vi "HAPS_PhaseSweep.vi"() -> ()   [LabVIEW 2023, in "HAPS.lvlib"]
uses:
  HAPS.lvlib
  MCU_Function.ctl
  set_ele.ctl
  HAPS_SerialPort.ctl
  HAPS_MCU_ELE_Func.ctl
panel:
  in  "comn_gain":i32=17
  in  "ele_gain":i32=35
  in  "File_note":string
  in  "Init?":bool
  out "Duration":dbl
  out "In-Phase : Phase(degree)":dbl[](graph)
  out "In-Phase : Gain(dB)":dbl[](graph)
  out "channel":i32
  out "chain_id":i32
  out "group":i32
  out "array_id":i32
  in  "Phase diff. Criteria":dbl format="%#_13g"
  in  "Tx/Rx":enum16{"Rx", "Tx"}(ring)=enum."Tx"
  in  "array_id (MCU index)":i32
  in  "MCU_UART_addr":refnum<visa-resource-name>="COM1"
  in  "Target(degree)":dbl format="%#_13g"
  in  "SweepPoints":i32=11
  in  "sParameter":i32=21
  in  "Stop_Freq(GHz)":dbl=39.5
  in  "Start_Freq(GHz)":dbl=38.5
  in  "VISA resource name":refnum<visa-resource-name>="TCPIP0::169.254.52.242::hislip0::INSTR"
  in  "HAPS_Equipment":enum16{"Keysight", "R&S"}(ring)
  # "HAPS_24x24_Phase_Sweep"
  # "VNA"
  # "Tx:35\nRx:22"
  # "DUT"
  # "4718.54"
  # "TCPIP0::192.168.1.31::hislip0::INSTR"
  # "Test Status"
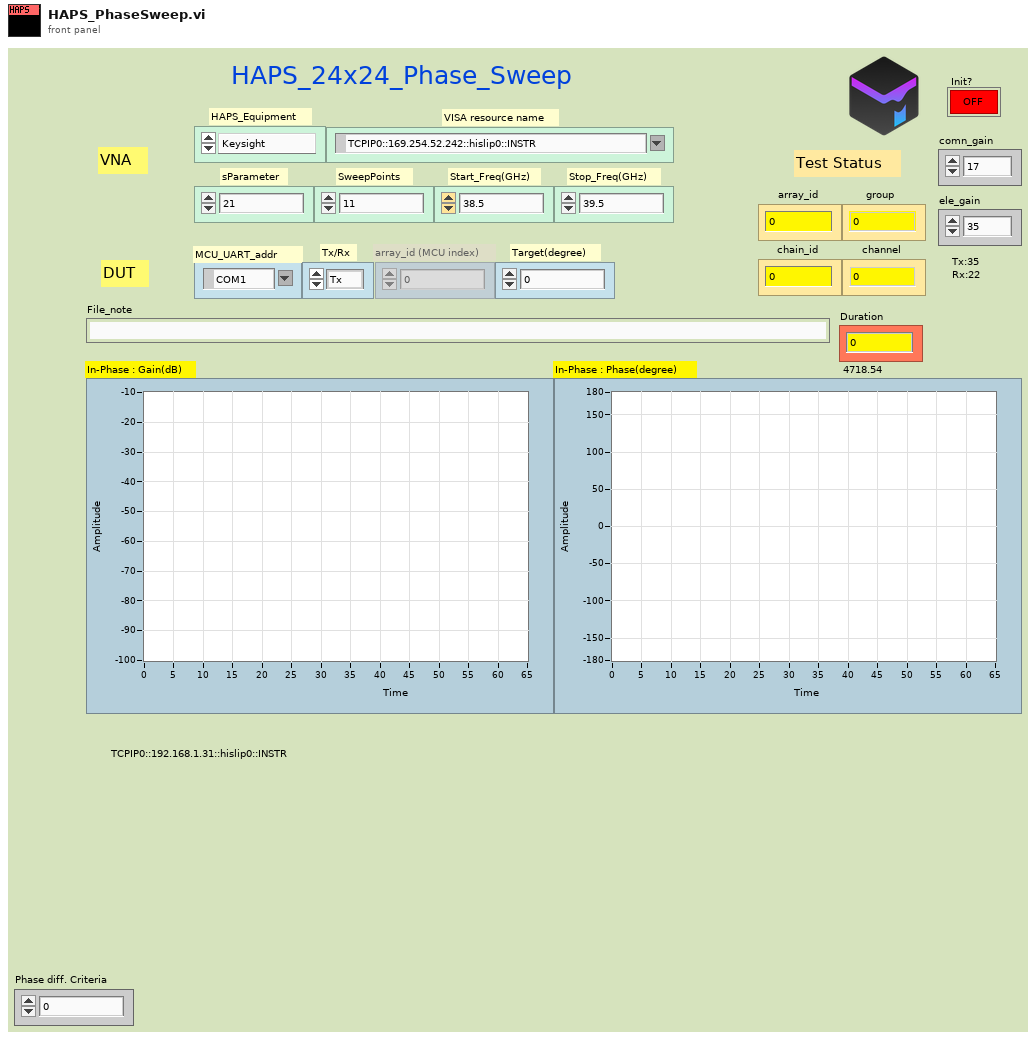
[diagram p1: front panel]
types:
  T1 = typedef "HAPS.lvlib/HAPS_SerialPort.ctl" = enum16{"Init", "Close", "CMD", "Flush"}
  T2 = typedef "HAPS.lvlib/HAPS_MCU_ELE_Func.ctl" = enum16{"array_init", "set_com_gain", "set_ch_gain_phase", "set_pd_range", "get_preamp_temp", "get_bfic_temp", "get_tx_pd", "ch_on", "ch_on_2", "ch_ctrl_all", "array_ctrl_src"}
  T3 = typedef "HAPS.lvlib/MCU_Function.ctl" = cluster{"Tx/Rx":enum16{"Rx", "Tx"}, "Enable?":enum16{"OFF", "On"}, "Source":enum16{"MCU", "ACU"}}
  T4 = typedef "HAPS.lvlib/set_ele.ctl" = cluster{"ch":i32, "chain_id":i32, "group":i32, "array_id":i32, "ele_phase":i32, "ele_gain":i32, "com_gain":i32, "pd_range":i32}
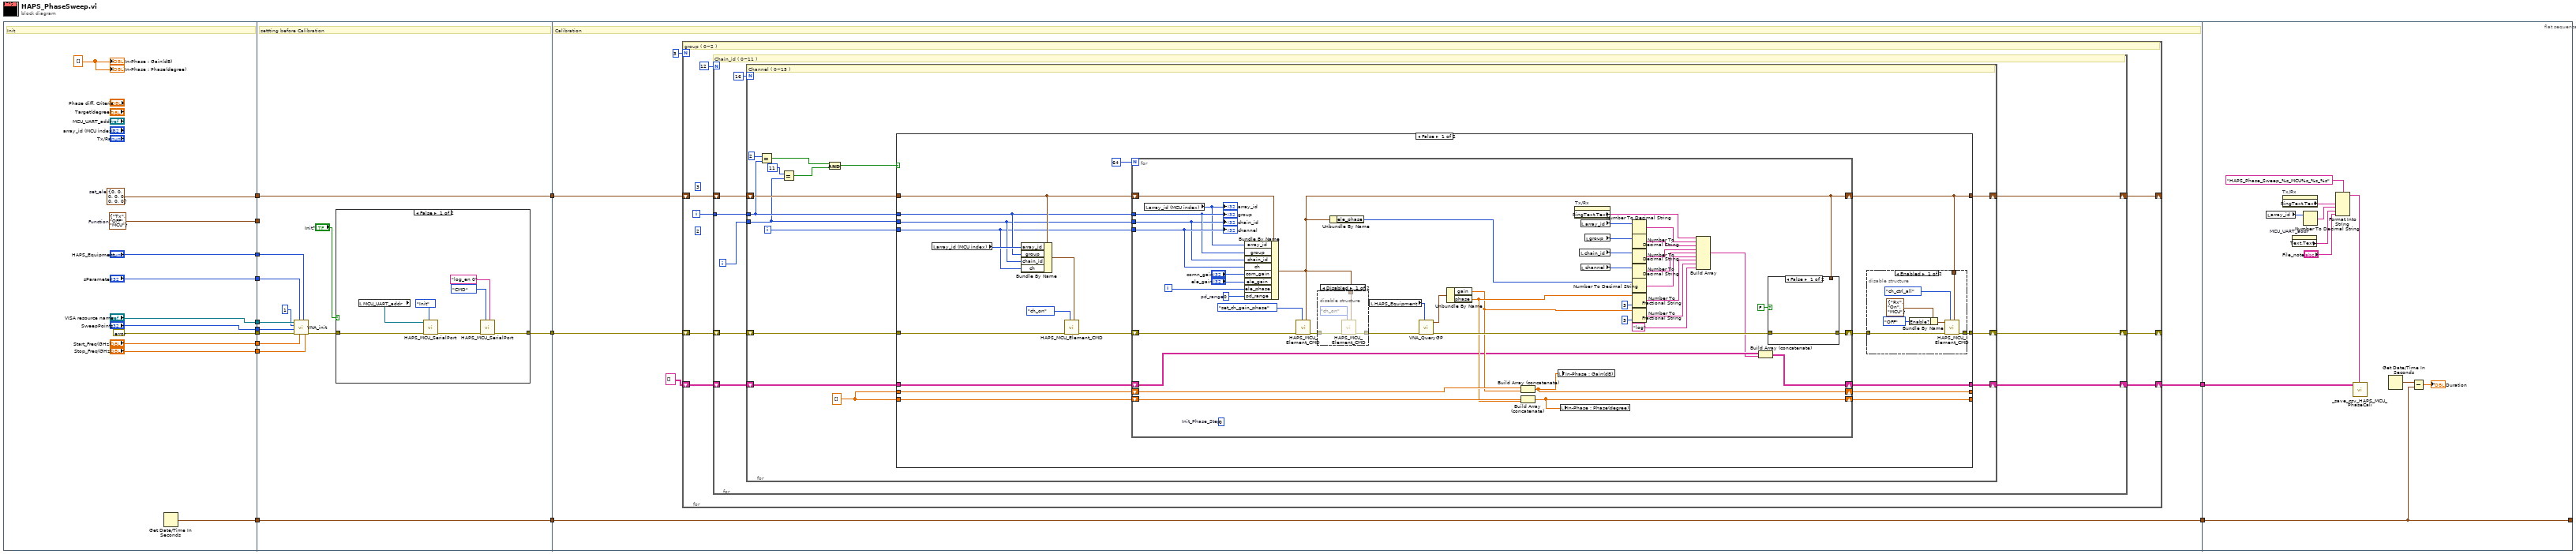
[diagram p0: block diagram]
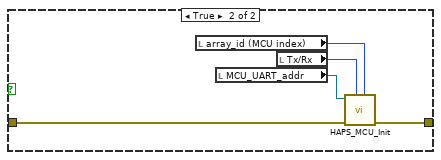
[diagram p2: hidden frame]
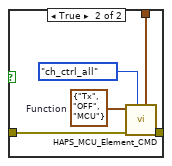
[diagram p5: hidden frame]
diagram:
  n1 = flat-sequence {
    tunnel: [w19] -> w15
    tunnel: [w26] -> w14
    tunnel: [errorcluster {"status"=FALSE, "code"=0, "source"=""} ("error in")] -> w12
    tunnel: ["sParameter"] -> w10
    tunnel: ["VISA resource name"] -> w9
    tunnel: ["Start_Freq(GHz)"] -> w8
    tunnel: ["Stop_Freq(GHz)"] -> w7
    tunnel: ["SweepPoints"] -> w6
    tunnel: ["HAPS_Equipment"] -> w5
    tunnel: [w16] -> w3
    tunnel: w15 -> [w39]
    tunnel: w14 -> [_]
    tunnel: [w39] -> w13
    tunnel: w12 -> [w38]
    tunnel: [w30] -> w11
    tunnel: w10 -> [w37]
    tunnel: w9 -> [w36]
    tunnel: w8 -> [w35]
    tunnel: w7 -> [w34]
    tunnel: w6 -> [w33]
    tunnel: w5 -> [w29]
    tunnel: [w28] -> w4
    tunnel: w3 -> [w28]
    tunnel: w13 -> [w56]
    tunnel: w11 -> [w57]
    tunnel: w4 -> [w53]
    tunnel: [w53] -> w2
    tunnel: [w52] -> w1
    tunnel: [w179] -> _
    tunnel: w2 -> [w179]
    tunnel: w1 -> [w181]
    frame #0 {
      w17 = dbl[] []
      w19 = T4 {"ch"=0, "chain_id"=0, "group"=0, "array_id"=0, "ele_phase"=0, "ele_gain"=0, "com_gain"=0, "pd_range"=0}  # set_ele
      w26 = T3 {"Tx/Rx"=enum."Tx", "Enable?"=enum."OFF", "Source"=enum."MCU"}  # Function
      # "Init"
      n2 = Get Date/Time In Seconds() -> (seconds since 1Jan1904=w16:timestamp)
      "In-Phase : Gain(dB)" <- w17
      "In-Phase : Phase(degree)" <- w17
    }
    frame #1 {
      # "settting before Calibration"
      n3 = call "VNA_init.vi"("Stop_Freq(GHz)"=w34, "HAPS_MCU_CMD"=w29, "Start_Freq(GHz)"=w35, "sParameter"=w37, "error in"=w38, "SweepPoints"=w33, "Mark no."=1, "VISA resource name"=w36) -> ("error out"=w31:errorcluster)  [unwired: 3 in]
      n4 = case shown="False" "Init?" {
        tunnel: w31 -> [w42 w51]
        tunnel: [w45 w50] -> w30
        frame False {
          n5 = local read "MCU_UART_addr"() -> (w40:refnum<visa-resource-name>)
          n6 = call "HAPS_MCU_SerialPort.vi"("HAPS_SerialPort_Func"=HAPS_SerialPort."Init", "error in"=w42, "VISA resource name"=w40) -> ("error out"=w43:errorcluster)  [unwired: 6 in, 2 out]
          n7 = call "HAPS_MCU_SerialPort.vi"("Command"="log_en 0", "HAPS_SerialPort_Func"=enum16{"Init", "Close", "CMD"}."CMD" ("HAPS_SerialPort"), "error in"=w43) -> ("error out"=w45:errorcluster)  [unwired: 6 in, 2 out]
        }
        frame True {
          n8 = local read "array_id (MCU index)"() -> (w48:i32)
          n9 = local read "MCU_UART_addr"() -> (w49:refnum<visa-resource-name>)
          n10 = local read "Tx/Rx"() -> (w47:enum16{"Rx", "Tx"})
          n11 = call "HAPS_MCU_Init.vi"("array_id"=w48, "Tx/Rx"=w47, "error in"=w51, "VISA resource name"=w49) -> ("error out"=w50:errorcluster)  [unwired: 7 in]
        }
      }
    }
    frame #2 {
      # "Calibration"
      n12 = for {
        N: 3 -> [_]
        shift-right: [w65] -> _
        shift-left: w56 -> [w61]
        shift-right: [w64] -> w52
        shift-left: string[][] [] -> [w60]
        shift-right: [w63] -> _
        shift-left: w57 -> [w62]
        i -> [w58]
        (unwired) 2
        (unwired) 3
        # "group ( 0~2 )"
        n13 = for {
          N: 12 -> [_]
          shift-right: [w73] -> w65
          shift-left: w61 -> [w70]
          shift-right: [w72] -> w64
          shift-left: w60 -> [w69]
          shift-right: [w66] -> w63
          shift-left: w62 -> [w71]
          tunnel: w58 -> [w68]
          i -> [w67]
          # "Chain_id ( 0~11 )"
          n14 = for {
            N: 16 -> [_]
            shift-right: [w86] -> w73
            shift-left: w70 -> [w89]
            shift-right: [w84] -> w72
            shift-left: w69 -> [w85]
            shift-right: [w87] -> w66
            shift-left: w71 -> [w88]
            tunnel: w68 -> [w83]
            tunnel: w67 -> [w75]
            i -> [w76]
            w77 = dbl[] []
            # "Channel ( 0~15 )"
            n15 = Equal?(x=2, y=w83) -> (x = y?=w80:bool)
            n16 = Equal?(x=11, y=w75) -> (x = y?=w79:bool)
            n17 = And(x=w80, y=w79) -> (x .and. y?=w78:bool)
            n18 = case shown="False" w78 {
              tunnel: w89 -> [w100 w173]
              tunnel: w76 -> [w97 _]
              tunnel: w88 -> [w94 w172]
              tunnel: w83 -> [w99 _]
              tunnel: w75 -> [w98 _]
              tunnel: w77 -> [w108 w175]
              tunnel: w77 -> [w107 w176]
              tunnel: [w106 w175] -> _
              tunnel: [w105 w176] -> _
              tunnel: [w91 w172] -> w87
              tunnel: [w90 w173] -> w86
              tunnel: w85 -> [w103 w174]
              tunnel: [w102 w174] -> w84
              frame False {
                n19 = local read "array_id (MCU index)"() -> (w101:i32)
                n20 = Bundle By Name(cluster=w100, "array_id"=w101, "group"=w99, "chain_id"=w98, "ch"=w97) -> (w93:T4)
                n21 = call "HAPS_MCU_Element_CMD.vi"("set_ele"=w93, "HAPS_MCU_ELE_Func."=HAPS_MCU_ELE_Func."ch_on", "error in"=w94) -> ("error out"=w95:errorcluster)  [unwired: 7 in, 1 out]
                n22 = for {
                  N: 64 -> [_]
                  tunnel: w97 -> [w159]
                  tunnel: w99 -> [w157]
                  tunnel: w98 -> [w156]
                  shift-right: [w132] -> w106
                  shift-left: w108 -> [w134]
                  shift-right: [w131] -> w105
                  shift-left: w107 -> [w133]
                  shift-right: [w128] -> w92
                  shift-left: w95 -> [w158]
                  shift-right: [w118] -> w90
                  shift-left: w100 -> [w160]
                  shift-right: [w122] -> w102
                  shift-left: w103 -> [w124]
                  i -> [w130]
                  w154 = 0  # pd_range
                  (unwired) 0  # Init_Phase_Step
                  n23 = local read "array_id (MCU index)"() -> (w152:i32)
                  "array_id" <- w152
                  n24 = Bundle By Name(cluster=w160, "array_id"=w152, "group"=w157, "chain_id"=w156, "ch"=w159, "com_gain"="comn_gain", "ele_gain"="ele_gain", "ele_phase"=w130, "pd_range"=w154) -> (w118:T4)
                  n25 = call "HAPS_MCU_Element_CMD.vi"("set_ele"=w118, "HAPS_MCU_ELE_Func."=HAPS_MCU_ELE_Func."set_ch_gain_phase", "error in"=w158) -> ("error out"=w120:errorcluster)  [unwired: 7 in, 1 out]
                  n26 = disable-structure shown="Disabled" {
                    disable-tunnel: w120 -> [w164 w165]
                    disable-tunnel: [w163 w165] -> w119
                    disable-tunnel: w118 -> [w161 _]
                    frame Disabled {
                      n27 = call "HAPS_MCU_Element_CMD.vi"("set_ele"=w161, "HAPS_MCU_ELE_Func."=HAPS_MCU_ELE_Func."ch_on", "error in"=w164) -> ("error out"=w163:errorcluster)  [unwired: 7 in, 1 out]
                    }
                    frame Enabled {
                    }
                  }
                  n28 = Unbundle By Name(w118) -> ("ele_phase"=w127:i32)
                  n29 = local read "HAPS_Equipment"() -> (w136:enum16{"Keysight", "R&S"})
                  n30 = call "VNA_QueryGP.vi"("HAPS_Equipment"=w136, "error in"=w119) -> ("error out"=w129:errorcluster, "queryMarker"=w135:cluster{"gain":dbl, "phase":dbl})  [unwired: 8 in]
                  n31 = Unbundle By Name(w135) -> ("gain"=w125:dbl, "phase"=w126:dbl)
                  n32 = Build Array (concatenate)(w133, w126) -> (w131:dbl[])
                  n33 = Build Array (concatenate)(w134, w125) -> (w132:dbl[])
                  n34 = local write "In-Phase : Gain(dB)"(w132) -> ()
                  n35 = local write "In-Phase : Phase(degree)"(w131) -> ()
                  n36 = property on="Tx/Rx" class="Enum (strict)"() -> ("RingText.Text"=w141:string)  [unwired: 2 in, 2 out]
                  n37 = local read "chain_id"() -> (w138:i32)
                  n38 = local read "array_id"() -> (w140:i32)
                  n39 = local read "channel"() -> (w137:i32)
                  n40 = local read "group"() -> (w139:i32)
                  n41 = Number To Decimal String(number=w140) -> (decimal integer string=w142:string)  [unwired: 1 in]
                  n42 = Number To Decimal String(number=w139) -> (decimal integer string=w143:string)  [unwired: 1 in]
                  n43 = Number To Decimal String(number=w138) -> (decimal integer string=w144:string)  [unwired: 1 in]
                  n44 = Number To Decimal String(number=w137) -> (decimal integer string=w145:string)  [unwired: 1 in]
                  n45 = Number To Decimal String(number=w127) -> (decimal integer string=w146:string)  [unwired: 1 in]
                  n46 = Number To Fractional String(number=w126, precision (6)=i16 3) -> (F-format string=w149:string)  [unwired: 2 in]
                  n47 = Number To Fractional String(number=w125, precision (6)=i16 3) -> (F-format string=w150:string)  [unwired: 2 in]
                  n48 = Build Array(w141, w142, w143, w144, w145, w146, w149, w150, "log") -> (w123:string[])
                  n49 = Build Array (concatenate)(w124, w123) -> (w122:string[][])
                  n50 = case shown="False" FALSE {
                    tunnel: w129 -> [w166 w169]
                    tunnel: [w166 w168] -> w128
                    tunnel: w118 -> [_ w167]
                    frame False {
                    }
                    frame True {
                      w171 = T3 {"Tx/Rx"=enum."Tx", "Enable?"=enum."OFF", "Source"=enum."MCU"}  # Function
                      n51 = call "HAPS_MCU_Element_CMD.vi"("set_ele"=w167, "HAPS_MCU_ELE_Func."=HAPS_MCU_ELE_Func."ch_ctrl_all", "error in"=w169, "Function"=w171) -> ("error out"=w168:errorcluster)  [unwired: 6 in, 1 out]
                    }
                  }
                  "group" <- w157
                  "chain_id" <- w156
                  "channel" <- w159
                }
                n52 = disable-structure shown="Enabled" {
                  disable-tunnel: w92 -> [w115 w116]
                  disable-tunnel: [w114 w116] -> w91
                  disable-tunnel: w90 -> [w109 _]
                  frame Enabled {
                    n53 = Bundle By Name(cluster=T3 {"Tx/Rx"=enum."Rx", "Enable?"=enum."On", "Source"=enum."MCU"} ("Function"), "Enable?"=enum16{"OFF", "On"}."OFF") -> (w111:T3)
                    n54 = call "HAPS_MCU_Element_CMD.vi"("set_ele"=w109, "HAPS_MCU_ELE_Func."=HAPS_MCU_ELE_Func."ch_ctrl_all", "error in"=w115, "Function"=w111) -> ("error out"=w114:errorcluster)  [unwired: 6 in, 1 out]
                  }
                  frame Disabled {
                  }
                }
              }
              frame True {
              }
            }
          }
        }
      }
    }
    frame #3 {
      n55 = local read "array_id"() -> (w184:i32)
      n56 = property on="Tx/Rx" class="Enum (strict)"() -> ("RingText.Text"=w183:string)  [unwired: 2 in, 2 out]
      n57 = property on="MCU_UART_addr" class="VISAName"() -> ("Text.Text"=w187:string)  [unwired: 2 in, 2 out]
      n58 = Number To Decimal String(number=w184) -> (decimal integer string=w185:string)  [unwired: 1 in]
      n59 = Format Into String(format string="HAPS_Phase_Sweep_%s_MCU%s_%s_%s", w183, w185, w187, "File_note") -> (resulting string=w186:string)  [unwired: 2 in, 1 out]
      n60 = call "_save_csv_HAPS_MCU_PhaseCali.vi"("NoteName"=w186, "array in"=w181) -> ()  [unwired: 9 in, 1 out]
      n61 = Get Date/Time In Seconds() -> (seconds since 1Jan1904=w180:timestamp)
      n62 = Subtract(x=w180, y=w179) -> (x-y=→"Duration":dbl)
    }
  }
